vi "HTTPTest.vi"() -> ()   [LabVIEW 2019]
uses:
  <vilib>/httpClient/POSTBuffer.vi
  <vilib>/regexp/Match Regular Expression.xnode
  <vilib>/httpClient/LabVIEWHTTPClient.lvlib
panel:
  out "value 2":T1
  out "body 3":string
  out "headers 4":string
  out "whole match":string
  out "selection":bool
  out "output string":string
  out "value":cluster{"String":string}
  out "JSON string":string
  out "body 2":string
  out "headers 3":string
  out "headers 2":string
  out "body":string
  out "headers":string
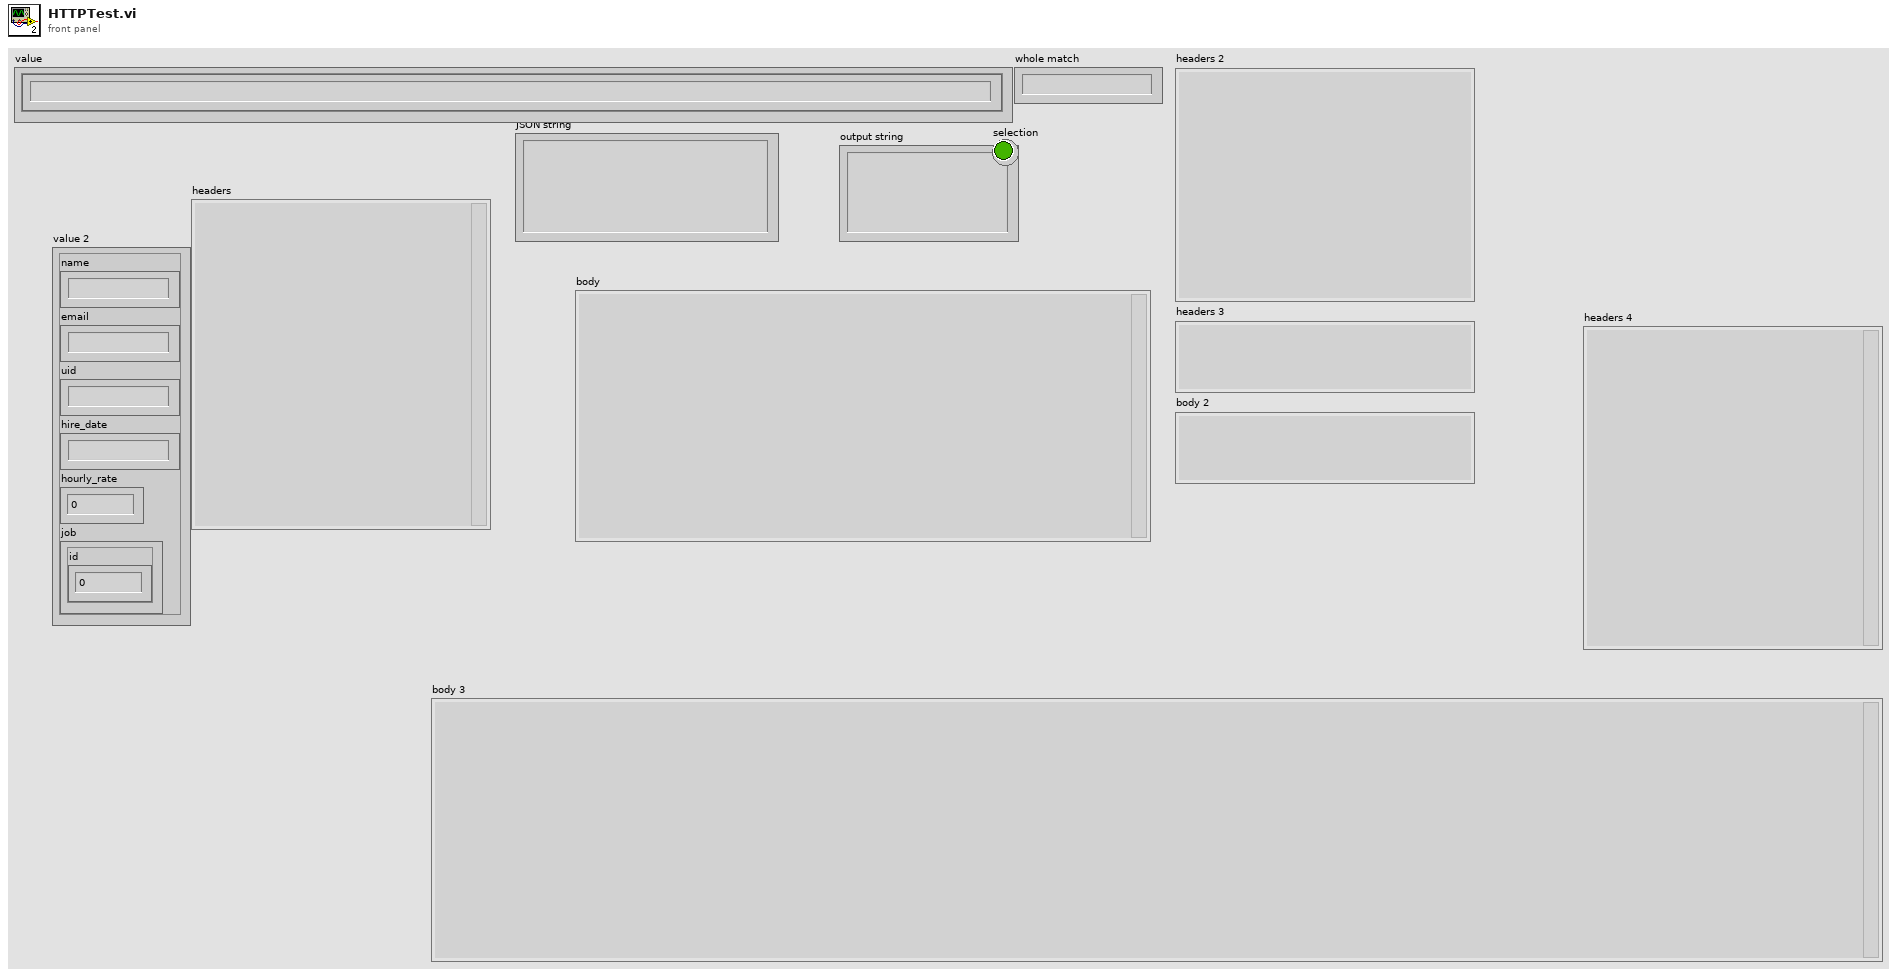
[diagram p1: front panel]
types:
  T1 = cluster{"name":string, "email":string, "uid":string, "hire_date":string, "hourly_rate":dbl, "job":cluster{"id":dbl}}
  T2 = typedef "LabVIEWHTTPClient.lvlib/ClientHandle.ctl" = refnum<k1>
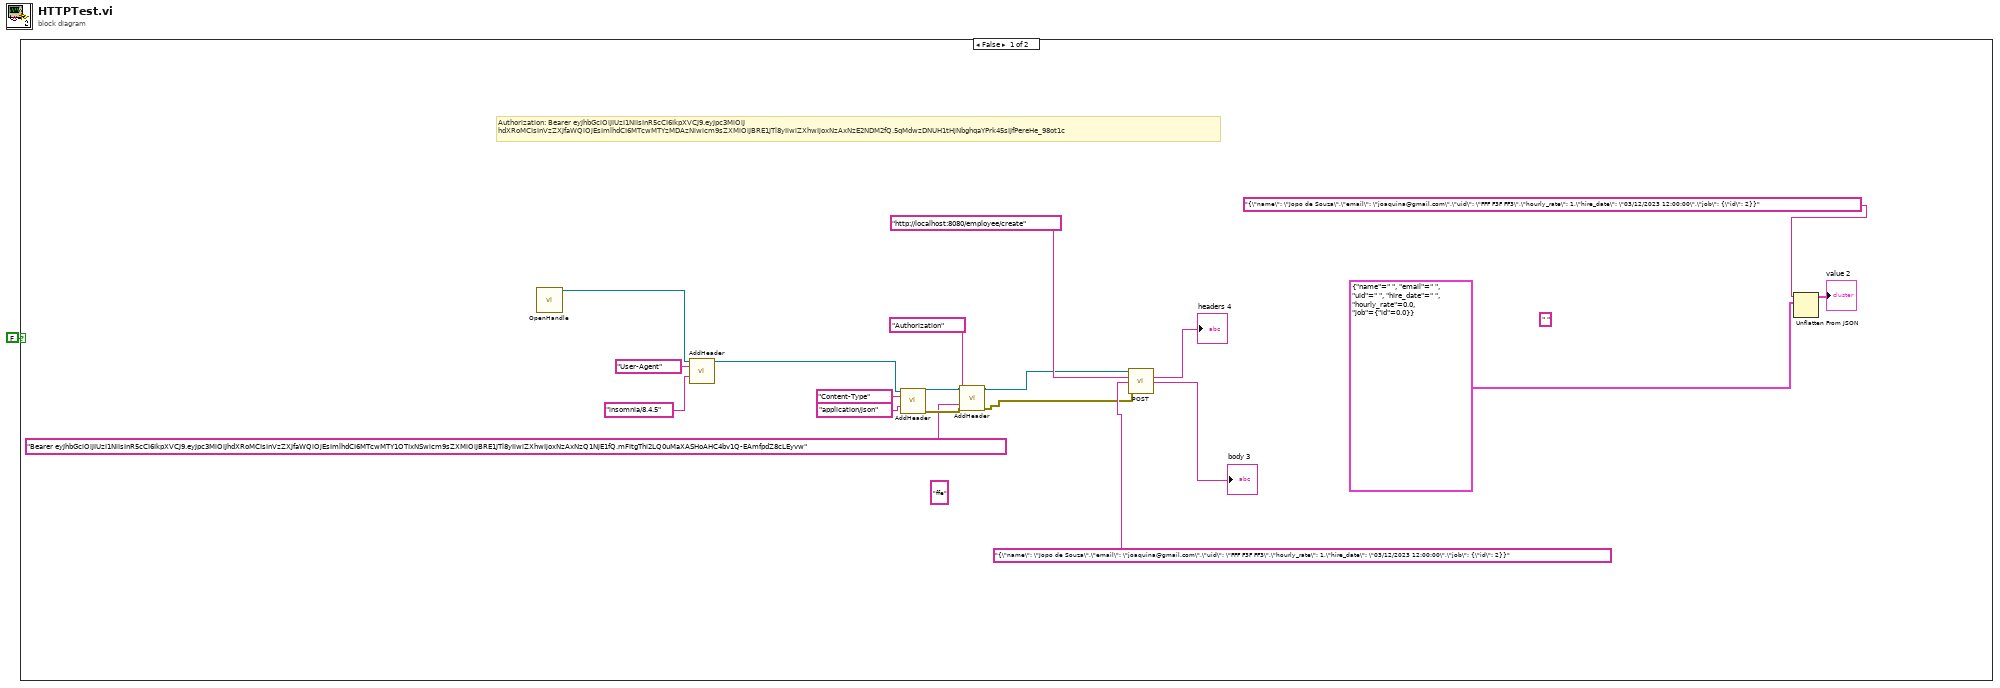
[diagram p0: block diagram]
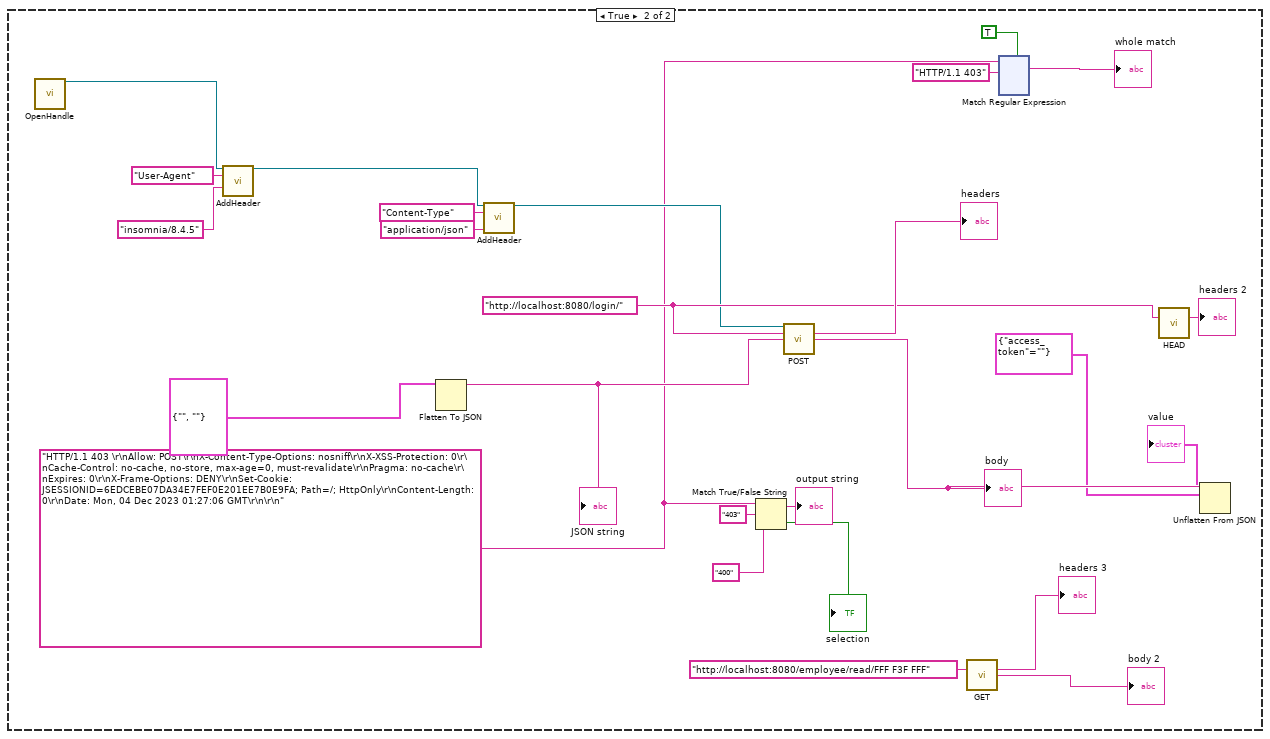
[diagram p2: hidden frame]
diagram:
  n1 = case shown="False" FALSE {
    frame False {
      (unwired) " "
      (unwired) "ffe" ("secret id")
      # "Authorization: Bearer eyJhbGciOiJIUzI1NiIsInR5cCI6IkpXVCJ9.eyJpc3MiOiJ\nhdXRoMCIsInVzZXJfaWQiOjEsImlhdCI6MTcwMTYzMDAzNiwicm9sZXMiOiJBRE1JTl8yIiwiZXhwIjoxNzAxNzE2NDM2fQ.5qMdwzDNUH1tHjNbghqaYPrk45sIJfPereHe_98ot1c"
      n2 = call <vilib>:"OpenHandle.vi"() -> ("client handle out"=w15:T2)  [unwired: 14 in, 1 out]
      n3 = call <vilib>:"AddHeader.vi"("client handle"=w15, "header"="User-Agent", "value"="insomnia/8.4.5") -> ("client handle out"=w20:T2)  [unwired: 11 in, 1 out]
      n4 = call <vilib>:"AddHeader.vi"("client handle"=w20, "header"="Content-Type", "value"="application/json") -> ("client handle out"=w8:T2, "error out"=w11:errorcluster)  [unwired: 11 in]
      n5 = call <vilib>:"AddHeader.vi"("client handle"=w8, "header"="Authorization", "value"="Bearer eyJhbGciOiJIUzI1NiIsInR5cCI6IkpXVCJ9.eyJpc3MiOiJhdXRoMCIsInVzZXJfaWQiOjEsImlhdCI6MTcwMTY1OTIxNSwicm9sZXMiOiJBRE1JTl8yIiwiZXhwIjoxNzAxNzQ1NjE1fQ.mFItgThi2LQ0uMaXASHoAHC4bv1Q-EAmfpdZ8cLEyvw", "error in (no error)"=w11) -> ("client handle out"=w9:T2, "error out"=w10:errorcluster)  [unwired: 10 in]
      n6 = call-poly <vilib>:"POST.vi"("client handle"=w9, "url"="http://localhost:8080/employee/create", "buffer"="{\"name\": \"Jopo de Souza\",\"email\": \"joaquina@gmail.com\",\"uid\": \"FFF F3F FF3\",\"hourly_rate\": 1,\"hire_date\": \"03/12/2023 12:00:00\",\"job\": {\"id\": 2}}" ("url"), "error in (no error)"=w10) -> ("headers"=→"headers 4":string, "body"=→"body 3":string)  [unwired: 8 in, 2 out]
      n7 = Unflatten From JSON(JSON string="{\"name\": \"Jopo de Souza\",\"email\": \"joaquina@gmail.com\",\"uid\": \"FFF F3F FF3\",\"hourly_rate\": 1,\"hire_date\": \"03/12/2023 12:00:00\",\"job\": {\"id\": 2}}", type and defaults=T1 {"name"=" ", "email"=" ", "uid"=" ", "hire_date"=" ", "hourly_rate"=0.0, "job"={"id"=0.0}}) -> (value=→"value 2":T1)  [unwired: 5 in, 1 out]
    }
    frame True {
      w24 = "HTTP/1.1 403 \r\nAllow: POST\r\nX-Content-Type-Options: nosniff\r\nX-XSS-Protection: 0\r\nCache-Control: no-cache, no-store, max-age=0, must-revalidate\r\nPragma: no-cache\r\nExpires: 0\r\nX-Frame-Options: DENY\r\nSet-Cookie: JSESSIONID=6EDCEBE07DA34E7FEF0E201EE7B0E9FA; Path=/; HttpOnly\r\nContent-Length: 0\r\nDate: Mon, 04 Dec 2023 01:27:06 GMT\r\n\r\n" ("string")
      w45 = "http://localhost:8080/login/" ("url")
      n8 = call <vilib>:"OpenHandle.vi"() -> ("client handle out"=w32:T2)  [unwired: 14 in, 1 out]
      n9 = call <vilib>:"AddHeader.vi"("client handle"=w32, "header"="User-Agent", "value"="insomnia/8.4.5") -> ("client handle out"=w35:T2)  [unwired: 11 in, 1 out]
      n10 = Flatten To JSON(anything=cluster{"login":string, "password":string} {"login"="", "password"=""}) -> (JSON string=w40:string)  [unwired: 2 in, 1 out]
      "JSON string" <- w40
      n11 = call <vilib>:"AddHeader.vi"("client handle"=w35, "header"="Content-Type", "value"="application/json") -> ("client handle out"=w38:T2)  [unwired: 11 in, 1 out]
      n12 = Match True/False String(2:"400" ("false string"), 3:"403" ("true string"), 4:w24) -> (0:→"selection":bool, 1:→"output string":string)
      n13 = call-poly <vilib>:"POST.vi"("client handle"=w38, "url"=w45, "buffer"=w40) -> ("headers"=→"headers":string, "body"=w31:string)  [unwired: 9 in, 2 out]
      "body" <- w31
      n14 = call <vilib>:"GET.vi"("url"="http://localhost:8080/employee/read/FFF F3F FFF") -> ("headers"=→"headers 3":string, "body"=→"body 2":string)  [unwired: 11 in, 2 out]
      n15 = xnode "Match Regular Expression"("input string"=w24, "regular expression"="HTTP/1.1 403", "multiline? (F)"=TRUE) -> ("whole match"=→"whole match":string)  [unwired: 3 in, 4 out]
      n16 = call <vilib>:"HEAD.vi"("url"=w45) -> ("headers"=→"headers 2":string)  [unwired: 12 in, 2 out]
      n17 = Unflatten From JSON(JSON string=w31, type and defaults=cluster{"access_token":string} {"access_token"=""}) -> (value=→"value":cluster{"access_token":string})  [unwired: 5 in, 1 out]
    }
  }
